vi "Configure Remote Trace Events.vi"(4 "Remote/Local (On)":bool=TRUE, 5 "Duration (On)":bool=TRUE, 6 "Connection (On)":bool=TRUE, 7 "Error (On)":bool=TRUE, 8 "error in (no error)":errorcluster, 9 "Output (On)":bool=TRUE, 10 "Input (On)":bool=TRUE, 11 "VISA resource name":refnum<visa-resource-name>) -> (0 "error out":errorcluster, 3 "VISA resource name out":refnum<visa-resource-name>)   [LabVIEW 2020, in "Rohde&Schwarz CMXP Base.lvlib"]
doc: "Selects which types of events are reported in the trace log.\n\nAttribute:\n-\n\nRemote-control command:\n[CONFigure:]BASE:RTRace:EVENts"
uses:
  <instrlib>/Rohde&Schwarz CMXP Base/Rohde&Schwarz CMXP Base.lvlib
  <instrlib>/Rohde&Schwarz CMXP Base/Private/rsidr_core.llb/rsidr_core.lvlib
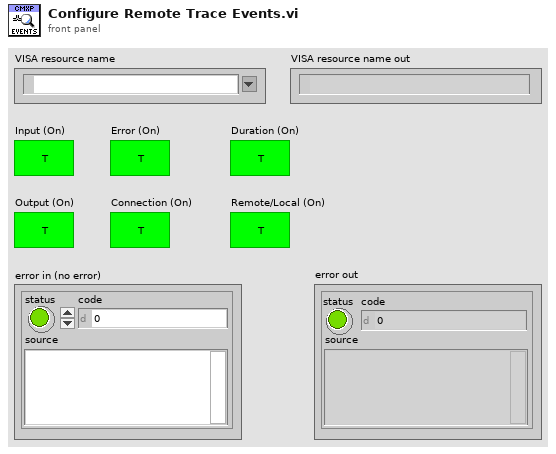
[diagram p1: front panel]
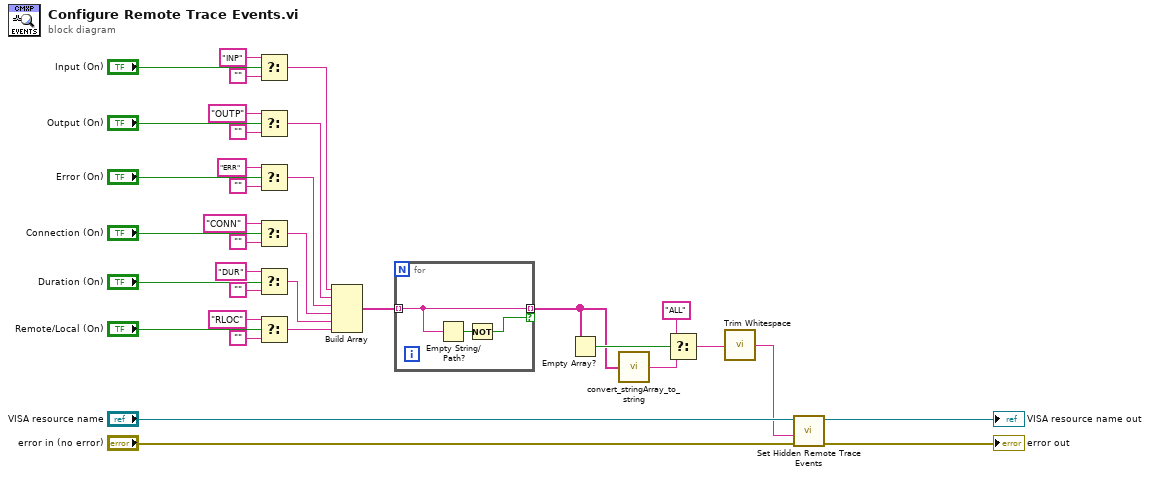
[diagram p0: block diagram]
diagram:
  n1 = Select(t="INP", s="Input (On)", f="" ("Empty String Constant")) -> (s? t:f=w23:string)
  n2 = Select(t="OUTP", s="Output (On)", f="" ("Empty String Constant")) -> (s? t:f=w22:string)
  n3 = Select(t="ERR", s="Error (On)", f="" ("Empty String Constant")) -> (s? t:f=w21:string)
  n4 = Select(t="CONN", s="Connection (On)", f="" ("Empty String Constant")) -> (s? t:f=w20:string)
  n5 = Select(t="DUR", s="Duration (On)", f="" ("Empty String Constant")) -> (s? t:f=w19:string)
  n6 = Select(t="RLOC", s="Remote/Local (On)", f="" ("Empty String Constant")) -> (s? t:f=w18:string)
  n7 = Build Array(w23, w22, w21, w20, w19, w18) -> (w6:string[])
  n8 = for {
    tunnel: w6 -> [w38] mode=indexing
    tunnel: [w38] -> w3 mode=indexing if=w36
    n9 = Empty String/Path?(string/path=w38) -> (empty?=w37:bool)
    n10 = Not(x=w37) -> (.not. x?=w36:bool)
  }
  n11 = Empty Array?(array=w3) -> (empty?=w5:bool)
  n12 = call <instrlib>:"convert_stringArray_to_string.vi"("string array in"=w3) -> ("string out"=w2:string)  [unwired: 4 in]
  n13 = Select(t="ALL", s=w5, f=w2) -> (s? t:f=w1:string)
  n14 = call <vilib>:"Trim Whitespace.vi"("string"=w1) -> ("trimmed string"=w7:string)  [unwired: 1 in]
  n15 = call "Set Hidden Remote Trace Events"("error in (no error)"="error in (no error)", "Hidden Remote Trace Events ()"=w7, "instrument handle"="VISA resource name") -> ("error out"=→"error out":errorcluster, "instrument handle out"=→"VISA resource name out":refnum<visa-resource-name>)  [unwired: 7 in]
